vi "Traverse_setup_tl.glob.vi"() -> ()   [LabVIEW 2010]
uses:
  Custom Controls/Axis_pos_cluster_tl.ctl
  Custom Controls/Axis_Control_tl.ctl
panel:
  in  "Stop Pressed?":bool
  out "Mac start pos":dbl format="%.5f"
  out "PRO-J start pos":i32
  in  "AXIS":T1 items=["Spare 0", "X", "Y", "Z", "THETA", "PHI", "Spare 6"]
  out "PULSES/mm":dbl format="%.2f"
  out "Current Position":dbl format="%.5f"
  in  "CURRENT POSITIONS":T2[](array[typedef])=[{"axis"="X", "mac position"=0.0}, {"axis"="Y", "mac position"=0.0}, {"axis"="Z", "mac position"=0.0}, {"axis"="PHI", "mac position"=0.0}, {"axis"="THETA", "mac position"=0.0}] {"mac position" format="%.5f"}
  in  "CHANNEL PARAMETERS":string[][](table)=[["NAME", "CARD", "FACTOR", "", "FFSCAL", "KP", "KI", "KD", "MAXERR", "MAXTIM", "WINDOW", "WINDOW TIM", "MAXVEL", "MAXACC", "", "", "", "FVEL", "FACC", "JOGVEL", "JOGACC", "HOMVEL", "HOMACC", "HOME FLAG", "HOMPOS", "FWDLIM", "REVLIM", "", "", ""], ["DEFAULT", "", "", "", "400000", "40", "50", "9000", "8000", "100", "10", "010", "400000", "1000000", "", "", "", "64000", "20000", "2000", "20000", "2000", "20000", "RC", "0", "1000000", "-1000000", "", "", ""], ["X", "1", "800", "", "400000", "40", "50", "9000", "8000", "100", "10", "010", "400000", "1000000", "", "", "", "64000", "20000", "2000", "20000", "2000", "20000", "RC", "0", "1000000", "-1000000", "", "", ""], ["Z", "2", "800", "", "400000", "40", "50", "9000", "8000", "100", "10", "010", "400000", "1000000", "", "", "", "30000", "20000", "2000", "20000", "10000", "20000", "RC", "0", "1000000", "-1000000", "", "", ""], ["Y", "3", "-1333.3333333", "", "400000", "40", "50", "9000", "8000", "100", "10", "010", "400000", "1000000", "", "", "", "64000", "20000", "2000", "20000", "2000", "20000", "RC", "0", "1000000", "-1000000", "", "", ""], ["PHI", "4", "34.184615", "", "400000", "8", "12", "20000", "8000", "100", "10", "010", "10000", "4000", "", "", "", "200", "2000", "200", "2000", "200", "2000", "RC", "0", "1000000", "-1000000", "", "", ""], ["THETA", "5", "11.11111", "", "400000", "40", "50", "9000", "8000", "100", "10", "010", "400000", "1000000", "", "", "", "64000", "20000", "2000", "20000", "2000", "20000", "RC", "0", "1000000", "-1000000", "", "", ""], ["", "", "", "", "", "", "", "", "", "", "", "", "", "", "", "", "", "", "", "", "", "", "", "", "", "", "", "", "", ""], ["", "", "", "", "", "", "", "", "", "", "", "", "", "", "", "", "", "", "", "", "", "", "", "", "", "", "", "", "", ""], ["", "", "", "", "", "", "", "", "", "", "", "", "", "", "", "", "", "", "", "", "", "", "", "", "", "", "", "", "", ""], ["", "", "", "", "", "", "", "", "", "", "", "", "", "", "", "", "", "", "", "", "", "", "", "", "", "", "", "", "", ""], ["", "", "", "", "", "", "", "", "", "", "", "", "", "", "", "", "", "", "", "", "", "", "", "", "", "", "", "", "", ""], ["", "", "", "", "", "", "", "", "", "", "", "", "", "", "", "", "", "", "", "", "", "", "", "", "", "", "", "", "", ""], ["", "", "", "", "", "", "", "", "", "", "", "", "", "", "", "", "", "", "", "", "", "", "", "", "", "", "", "", "", ""], ["", "", "", "", "", "", "", "", "", "", "", "", "", "", "", "", "", "", "", "", "", "", "", "", "", "", "", "", "", ""], ["", "", "", "", "", "", "", "", "", "", "", "", "", "", "", "", "", "", "", "", "", "", "", "", "", "", "", "", "", ""]]
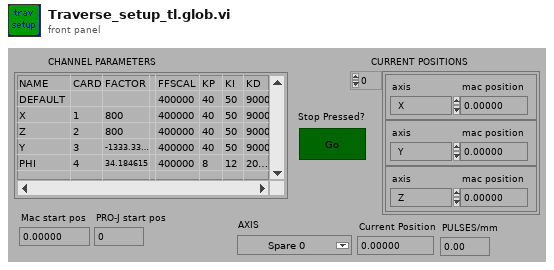
[diagram p1: front panel]
types:
  T1 = typedef "Axis_Control_tl.ctl" = u16
  T2 = typedef "Axis_pos_cluster_tl.ctl" = cluster{"axis":string, "mac position":dbl}
diagram:
